vi "MInda Welcome Screen.vi"(1 "error in":errorcluster) -> (0 "error out":errorcluster)   [LabVIEW 2017]
panel:
  # "REPORT GENERATION SYSTEM"
  # "Developed By\n\nNIVISION SYSTEMS Pune."
  # "Contact:-- 09325640282.\nEmail:-- sales@nivision.in\nwww.nivision.in"
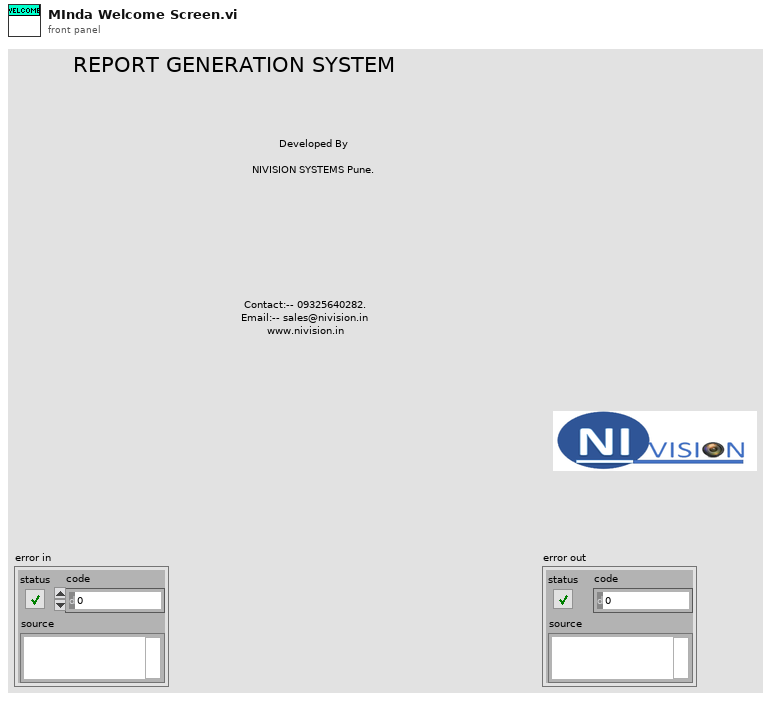
[diagram p1: front panel]
types:
  T1 = enum32{"Invalid", "Standard", "Closed", "Hidden", "Minimized", "Maximized"}
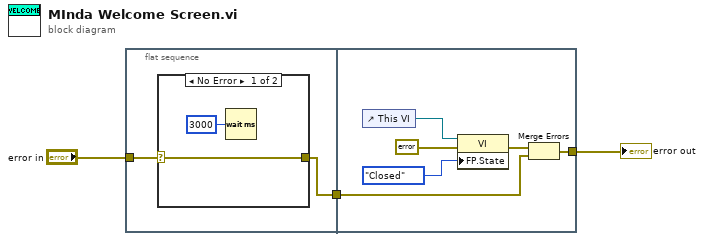
[diagram p0: block diagram]
diagram:
  n1 = flat-sequence {
    tunnel: [w4] -> w2
    tunnel: "error in" -> [w5]
    tunnel: [w10] -> w3
    tunnel: w2 -> [w9]
    frame #0 {
      n2 = case shown="No Error" w5 {
        selector: w5 -> [w6 w8]
        tunnel: [w6 w8] -> w4
        frame No Error {
          n3 = Wait (ms)(milliseconds to wait=u32 3000) -> ()  [unwired: 1 out]
        }
        frame Error {
        }
      }
    }
    frame #1 {
      n4 = control-ref of="This VI"() -> (w14:refnum<vi>)
      n5 = property class="VI"(reference=w14, error in=errorcluster {"status"=FALSE, "code"=0, "source"=""} ("error in (no error)"), "FP.State"=T1."Closed" ("Front Panel Window:State")) -> (error out=w12:errorcluster)  [unwired: 1 out]
      n6 = Merge Errors(w12, w9) -> (w10:errorcluster)
    }
  }
  "error out" <- w3
